vi "Partial Tokens.vi"(8 "Error In":errorcluster, 11 "All Tokens":refnum<class "Abstract.lvclass">[](array[class])) -> (0 "Error Out":errorcluster, 3 "Partial Tokens":refnum<class "Partial.lvclass">[](array[class]))   [LabVIEW 2018, in "Toolkit.lvlib" / "Compiler.lvclass"]
uses:
  Compiler.lvclass
  Tokens/Abstract/Abstract.lvclass
  Tokens/Partial/Partial.lvclass
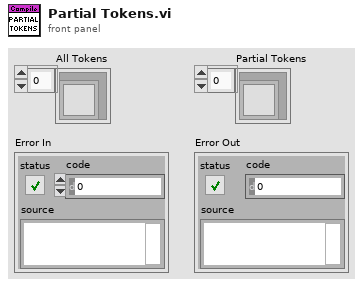
[diagram p1: front panel]
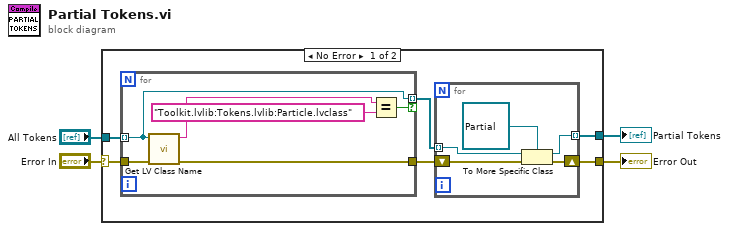
[diagram p0: block diagram]
diagram:
  n1 = case shown="No Error" "Error In" {
    selector: "Error In" -> [w5 w22]
    tunnel: "All Tokens" -> [w9 _]
    tunnel: [w8 w22] -> w3
    tunnel: [w6 _] -> w2
    frame No Error {
      n2 = for {
        tunnel: w9 -> [w17] mode=indexing
        tunnel: w5 -> [w21]
        tunnel: [w20] -> w10
        tunnel: [w17] -> w7 mode=indexing if=w16
        n3 = call <vilib>:"Get LV Class Name.vi"("error in (no error)"=w21, "object"=w17) -> ("error out"=w20:errorcluster, "class name"=w19:string)  [unwired: 8 in]
        n4 = Equal?(x=w19, y="Toolkit.lvlib:Tokens.lvlib:Particle.lvclass") -> (x = y?=w16:bool)
      }
      n5 = for {
        shift-right: [w14] -> w8
        shift-left: w10 -> [w15]
        tunnel: w7 -> [w13] mode=indexing
        tunnel: [w11] -> w6 mode=indexing
        n6 = To More Specific Class(target class=refnum<class "Partial.lvclass"> refnum ("Toolkit.lvlib:Tokens.lvlib:Partial.lvclass"), reference=w13, error in=w15) -> (specific class reference=w11:refnum<class "Partial.lvclass">, error out=w14:errorcluster)
      }
    }
    frame Error {
    }
  }
  "Error Out" <- w3
  "Partial Tokens" <- w2
